vi "time string to time stamp.vi"(10 "time string example(16:15:00)":string) -> (2 "time stamp":timestamp)   [LabVIEW 2011]
uses:
  <vilib>/Utility/miscctls.llb/LVDateTimeRec.ctl
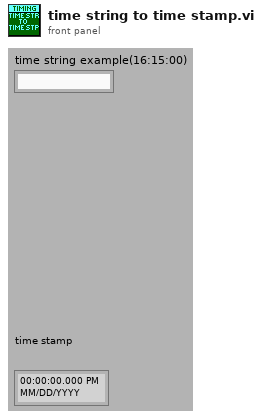
[diagram p1: front panel]
types:
  T1 = typedef "LVDateTimeRec.ctl" = cluster{"fractional second":dbl, "second":i32, "minute":i32, "hour":i32, "day of month":i32, "month":i32, "year":i32, "day of week":i32, "day of year":i32, "DST":i32}
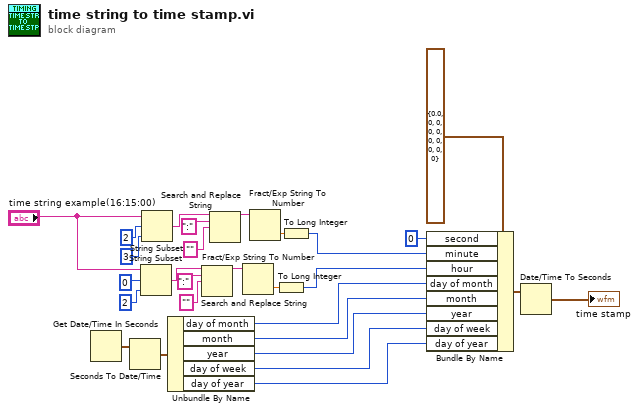
[diagram p0: block diagram]
diagram:
  n1 = Get Date/Time In Seconds() -> (seconds since 1Jan1904=w26:timestamp)
  n2 = Seconds To Date/Time(time stamp (now)=w26) -> (date time rec=w25:T1)  [unwired: 1 in]
  n3 = String Subset(string="time string example(16:15:00)", offset (0)=0, length (rest)=2 ("length (len. of substring)")) -> (substring=w16:string)
  n4 = String Subset(string="time string example(16:15:00)", offset (0)=2, length (rest)=3 ("length (len. of substring)")) -> (substring=w9:string)
  n5 = Unbundle By Name(w25) -> ("day of month"=w24:i32, "month"=w23:i32, "year"=w22:i32, "day of week"=w21:i32, "day of year"=w20:i32)
  n6 = Search and Replace String(input string=w16, search string=":" ("substring (\"\")"), replace string="" ("substring (\"\")")) -> (result string=w13:string)  [unwired: 5 in, 3 out]
  n7 = Search and Replace String(input string=w9, search string=":" ("substring (\"\")"), replace string="" ("substring (\"\")")) -> (result string=w6:string)  [unwired: 5 in, 3 out]
  n8 = Fract/Exp String To Number(string=w13) -> (number=w4:dbl)  [unwired: 3 in, 1 out]
  n9 = Fract/Exp String To Number(string=w6) -> (number=w5:dbl)  [unwired: 3 in, 1 out]
  n10 = To Long Integer(number=w4) -> (32bit integer=w2:i32)
  n11 = To Long Integer(number=w5) -> (32bit integer=w1:i32)
  n12 = Bundle By Name(cluster=T1 {"fractional second"=0.0, "second"=0, "minute"=0, "hour"=0, "day of month"=0, "month"=0, "year"=0, "day of week"=0, "day of year"=0, "DST"=0} ("date time rec"), "second"=0, "minute"=w1, "hour"=w2, "day of month"=w24, "month"=w23, "year"=w22, "day of week"=w21, "day of year"=w20) -> (w28:T1)
  n13 = Date/Time To Seconds(2:w28) -> (0:→"time stamp":timestamp)  [unwired: 1 in]
